vi "InitConfiguration.vi"(8 "error in":errorcluster) -> (0 "error out":errorcluster)   [LabVIEW 2012]
uses:
  <vilib>/Utility/config.llb/Read Key (U32).vi
  <vilib>/Utility/config.llb/Read Key (Double).vi
  GlobalVariables/GantnerParameters.vi
  <vilib>/Utility/config.llb/Read Key (String).vi
  GlobalVariables/PT02Parameters.vi
  GlobalVariables/PT03Parameters.vi
  <vilib>/Utility/config.llb/Read Key (I32).vi
  GlobalVariables/FT01Parameters.vi
  GlobalVariables/FT02Parameters.vi
  <vilib>/Utility/config.llb/Read Key (Boolean).vi
  GlobalVariables/SystemParameters.vi
  GlobalVariables/HardwarePresent.vi
  GlobalVariables/StabilizationSettings.vi
  <vilib>/Utility/config.llb/NI_LVConfig.lvlib
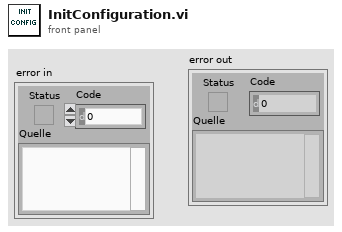
[diagram p1: front panel]
types:
  T1 = typedef "NI_LVConfig.lvlib/Config Data RefNum.ctl" = refnum<k1>
  T2 = typedef "ISMBUS_Module.ctl" = cluster{"ModuleAddress":i32, "ModuleKindIndex":i32, "ModuleKind":string, " Protocol":string, " BaudRate":i32, "CharFormat":string, "BaudRateIndex":i32, "FormatIndex":i32, "ProtocolIndex":i32, "Location":string, "SerialNumber":string, "Vendor":string, "HWRelease":string, "SWRelease":string, "ControllerType":string, "ChannelList":T3[], "ChannelCount":i32, " COM Port":i32}
  T3 = typedef "ISMBUS_Channel.ctl" = cluster{" Description":string, " ChannelKindIndex":i32, "ChannelFormatIndex":i32, " FieldLength":i32, "Precision":i32, "Unit":string, "Mode":i32}
  T4 = cluster{"Module":T2, "value":u32, "value":u32, "value":u32, "value":u32, "value":dbl}
  T5 = cluster{"value":u32, "value":string, "value":u32, "value":dbl, "value":u32}
  T6 = cluster{"value":u32, "value":i32, "value":i32, "value":dbl, "IDH":u8, "IDM":u8, "IDL":u8, "IDS":u8}
  T7 = cluster{"value":string, "value":string, "value":string, "value":bool}
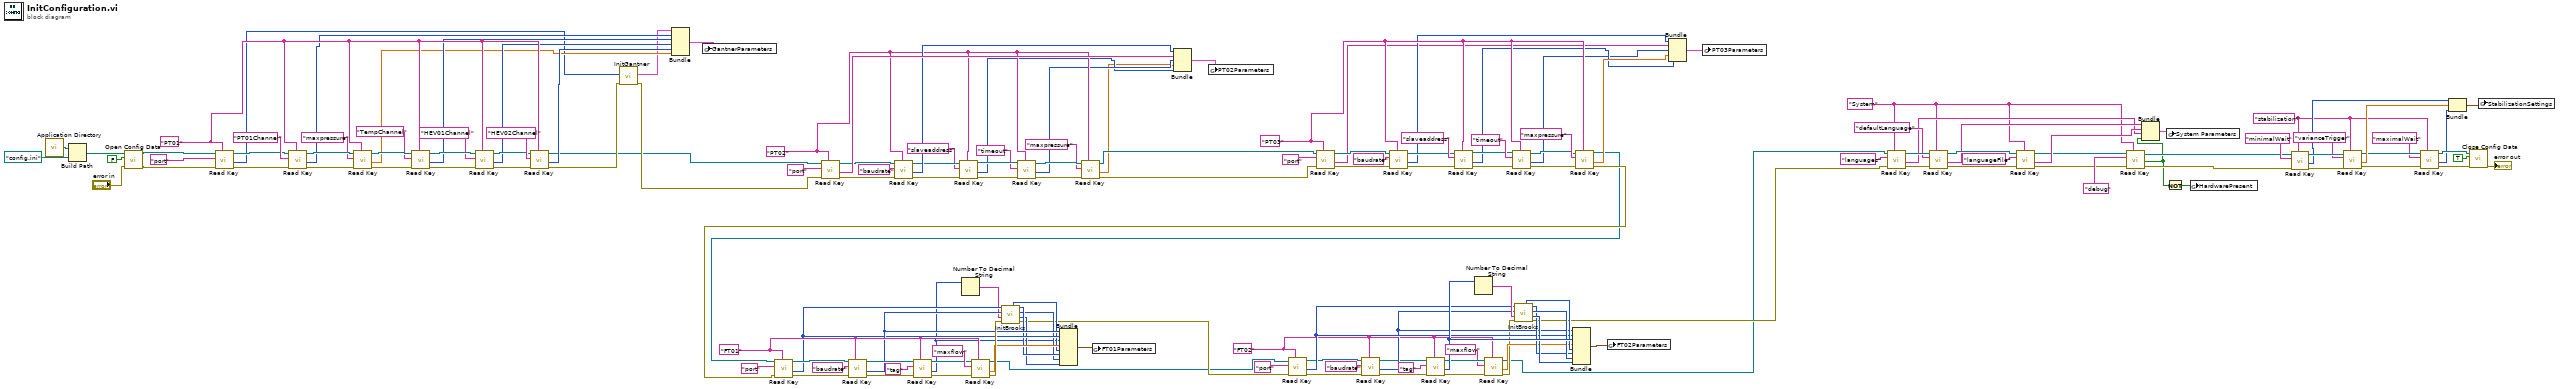
[diagram p0: block diagram]
diagram:
  w18 = "FT02" ("section")
  w40 = "FT01" ("section")
  w76 = "PT02" ("section")
  w108 = "PT01" ("section")
  w119 = "stabilization"
  w114 = "System" ("section")
  w124 = "PT03" ("section")
  n1 = call <vilib>:"Application Directory.vi"() -> ("Application Directory"=w158:path)
  n2 = Build Path(base path=w158, name or relative path=path "config.ini" ("default name")) -> (appended path=w159:path)
  n3 = call <vilib>:"Open Config Data.vi"("error in (no error)"="error in", "create file if necessary (T)"=FALSE ("create file if necessary? (T)"), "configuration file path"=w159) -> ("error out"=w89:errorcluster, "refnum"=w90:T1)  [unwired: 6 in, 1 out]
  n4 = call-poly <vilib>:"Read Key.vi"("section"=w108, "error in (no error)"=w89, "key"="port", "refnum"=w90) -> ("error out"=w102:errorcluster, "value"=w83:u32, "refnum out"=w103:T1)  [unwired: 4 in, 1 out]
  n5 = call-poly <vilib>:"Read Key.vi"("section"=w108, "error in (no error)"=w102, "key"="PT01Channel", "refnum"=w103) -> ("error out"=w107:errorcluster, "value"=w88:u32, "refnum out"=w106:T1)  [unwired: 4 in, 1 out]
  n6 = call-poly <vilib>:"Read Key.vi"("section"=w108, "error in (no error)"=w107, "key"="maxpressure", "refnum"=w106) -> ("error out"=w99:errorcluster, "value"=w84:dbl, "refnum out"=w100:T1)  [unwired: 4 in, 1 out]
  n7 = call-poly <vilib>:"Read Key.vi"("section"=w108, "error in (no error)"=w99, "key"="TempChannel", "refnum"=w100) -> ("error out"=w93:errorcluster, "value"=w87:u32, "refnum out"=w94:T1)  [unwired: 4 in, 1 out]
  n8 = call-poly <vilib>:"Read Key.vi"("section"=w108, "error in (no error)"=w93, "key"="HEV01Channel", "refnum"=w94) -> ("error out"=w95:errorcluster, "value"=w86:u32, "refnum out"=w96:T1)  [unwired: 4 in, 1 out]
  n9 = call-poly <vilib>:"Read Key.vi"("section"=w108, "error in (no error)"=w95, "key"="HEV02Channel", "refnum"=w96) -> ("error out"=w81:errorcluster, "value"=w85:u32, "refnum out"=w60:T1)  [unwired: 4 in, 1 out]
  n10 = call "InitGantner.vi"("error in"=w81, "Port"=w83) -> ("error out"=w61:errorcluster, "Module"=w82:T2)  [unwired: 8 in]
  n11 = Bundle("Module"=w82, "value"=w88, "value"=w87, "value"=w86, "value"=w85, "value"=w84) -> (w98:T4)  [unwired: 1 in]
  n12 = global write "GantnerParameters.vi" "GantnerParameters"(w98) -> ()
  n13 = call-poly <vilib>:"Read Key.vi"("section"=w76, "error in (no error)"=w61, "key"="port", "refnum"=w60) -> ("error out"=w70:errorcluster, "value"=w78:string, "refnum out"=w71:T1)  [unwired: 4 in, 1 out]
  n14 = call-poly <vilib>:"Read Key.vi"("section"=w76, "error in (no error)"=w70, "key"="baudrate", "refnum"=w71) -> ("error out"=w75:errorcluster, "value"=w77:u32, "refnum out"=w74:T1)  [unwired: 4 in, 1 out]
  n15 = call-poly <vilib>:"Read Key.vi"("section"=w76, "error in (no error)"=w75, "key"="slaveaddress", "refnum"=w74) -> ("error out"=w67:errorcluster, "value"=w55:u32, "refnum out"=w68:T1)  [unwired: 4 in, 1 out]
  n16 = call-poly <vilib>:"Read Key.vi"("section"=w76, "error in (no error)"=w67, "key"="timeout", "refnum"=w68) -> ("error out"=w64:errorcluster, "value"=w56:u32, "refnum out"=w65:T1)  [unwired: 4 in, 1 out]
  n17 = call-poly <vilib>:"Read Key.vi"("section"=w76, "error in (no error)"=w64, "key"="maxpressure", "refnum"=w65) -> ("error out"=w59:errorcluster, "value"=w54:dbl, "refnum out"=w58:T1)  [unwired: 4 in, 1 out]
  n18 = Bundle("value"=w77, "value"=w78, "value"=w56, "value"=w54, "value"=w55) -> (w66:T5)  [unwired: 1 in]
  n19 = global write "PT02Parameters.vi" "PT02Parameters"(w66) -> ()
  n20 = call-poly <vilib>:"Read Key.vi"("section"=w124, "error in (no error)"=w59, "key"="port", "refnum"=w58) -> ("error out"=w148:errorcluster, "value"=w79:string, "refnum out"=w147:T1)  [unwired: 4 in, 1 out]
  n21 = call-poly <vilib>:"Read Key.vi"("section"=w124, "error in (no error)"=w148, "key"="baudrate", "refnum"=w147) -> ("error out"=w143:errorcluster, "value"=w80:u32, "refnum out"=w144:T1)  [unwired: 4 in, 1 out]
  n22 = call-poly <vilib>:"Read Key.vi"("section"=w124, "error in (no error)"=w143, "key"="slaveaddress", "refnum"=w144) -> ("error out"=w151:errorcluster, "value"=w52:u32, "refnum out"=w150:T1)  [unwired: 4 in, 1 out]
  n23 = call-poly <vilib>:"Read Key.vi"("section"=w124, "error in (no error)"=w151, "key"="timeout", "refnum"=w150) -> ("error out"=w154:errorcluster, "value"=w51:u32, "refnum out"=w153:T1)  [unwired: 4 in, 1 out]
  n24 = call-poly <vilib>:"Read Key.vi"("section"=w124, "error in (no error)"=w154, "key"="maxpressure", "refnum"=w153) -> ("error out"=w6:errorcluster, "value"=w53:dbl, "refnum out"=w5:T1)  [unwired: 4 in, 1 out]
  n25 = call-poly <vilib>:"Read Key.vi"("section"=w40, "error in (no error)"=w6, "key"="port", "refnum"=w5) -> ("error out"=w46:errorcluster, "value"=w37:i32, "refnum out"=w45:T1)  [unwired: 4 in, 1 out]
  n26 = call-poly <vilib>:"Read Key.vi"("section"=w40, "error in (no error)"=w46, "key"="baudrate", "refnum"=w45) -> ("error out"=w41:errorcluster, "value"=w38:u32, "refnum out"=w42:T1)  [unwired: 4 in, 1 out]
  n27 = call-poly <vilib>:"Read Key.vi"("section"=w40, "error in (no error)"=w41, "key"="tag", "refnum"=w42) -> ("error out"=w49:errorcluster, "value"=w30:i32, "refnum out"=w48:T1)  [unwired: 4 in, 1 out]
  n28 = Number To Decimal String(number=w30) -> (decimal integer string=w29:string)  [unwired: 1 in]
  n29 = call-poly <vilib>:"Read Key.vi"("section"=w40, "error in (no error)"=w49, "key"="maxflow", "refnum"=w48) -> ("error out"=w39:errorcluster, "value"=w36:dbl, "refnum out"=w3:T1)  [unwired: 4 in, 1 out]
  n30 = call "InitBrooks.vi"("error in"=w39, "TAG"=w29, "Baud"=w38, "COM"=w37) -> ("error out"=w4:errorcluster, "IDS"=w32:u8, "IDL"=w33:u8, "IDM"=w34:u8, "IDH"=w35:u8)  [unwired: 3 in]
  n31 = Bundle("value"=w38, "value"=w37, "value"=w30, "value"=w36, "IDH"=w35, "IDM"=w34, "IDL"=w33, "IDS"=w32) -> (w31:T6)  [unwired: 1 in]
  n32 = global write "FT01Parameters.vi" "FT01Parameters"(w31) -> ()
  n33 = call-poly <vilib>:"Read Key.vi"("section"=w18, "error in (no error)"=w4, "key"="port", "refnum"=w3) -> ("error out"=w12:errorcluster, "value"=w21:i32, "refnum out"=w13:T1)  [unwired: 4 in, 1 out]
  n34 = call-poly <vilib>:"Read Key.vi"("section"=w18, "error in (no error)"=w12, "key"="baudrate", "refnum"=w13) -> ("error out"=w17:errorcluster, "value"=w20:u32, "refnum out"=w16:T1)  [unwired: 4 in, 1 out]
  n35 = call-poly <vilib>:"Read Key.vi"("section"=w18, "error in (no error)"=w17, "key"="tag", "refnum"=w16) -> ("error out"=w9:errorcluster, "value"=w27:i32, "refnum out"=w10:T1)  [unwired: 4 in, 1 out]
  n36 = Number To Decimal String(number=w27) -> (decimal integer string=w28:string)  [unwired: 1 in]
  n37 = call-poly <vilib>:"Read Key.vi"("section"=w18, "error in (no error)"=w9, "key"="maxflow", "refnum"=w10) -> ("error out"=w19:errorcluster, "value"=w22:dbl, "refnum out"=w1:T1)  [unwired: 4 in, 1 out]
  n38 = call "InitBrooks.vi"("error in"=w19, "TAG"=w28, "Baud"=w20, "COM"=w21) -> ("error out"=w2:errorcluster, "IDS"=w26:u8, "IDL"=w25:u8, "IDM"=w24:u8, "IDH"=w23:u8)  [unwired: 3 in]
  n39 = Bundle("value"=w20, "value"=w21, "value"=w27, "value"=w22, "IDH"=w23, "IDM"=w24, "IDL"=w25, "IDS"=w26) -> (w7:T6)  [unwired: 1 in]
  n40 = global write "FT02Parameters.vi" "FT02Parameters"(w7) -> ()
  n41 = Bundle("value"=w80, "value"=w79, "value"=w51, "value"=w53, "value"=w52) -> (w57:T5)  [unwired: 1 in]
  n42 = global write "PT03Parameters.vi" "PT03Parameters"(w57) -> ()
  n43 = call-poly <vilib>:"Read Key.vi"("section"=w114, "error in (no error)"=w2, "key"="languages" ("section"), "refnum"=w1) -> ("error out"=w139:errorcluster, "value"=w133:string, "refnum out"=w142:T1)  [unwired: 4 in, 1 out]
  n44 = call-poly <vilib>:"Read Key.vi"("section"=w114, "error in (no error)"=w139, "key"="defaultLanguage" ("section"), "refnum"=w142) -> ("error out"=w140:errorcluster, "value"=w135:string, "refnum out"=w141:T1)  [unwired: 4 in, 1 out]
  n45 = call-poly <vilib>:"Read Key.vi"("section"=w114, "error in (no error)"=w140, "key"="languageFile" ("section"), "refnum"=w141) -> ("error out"=w111:errorcluster, "value"=w134:string, "refnum out"=w109:T1)  [unwired: 4 in, 1 out]
  n46 = call-poly <vilib>:"Read Key.vi"("section"=w114, "error in (no error)"=w111, "key"="debug", "refnum"=w109) -> ("error out"=w115:errorcluster, "value"=w110:bool, "refnum out"=w116:T1)  [unwired: 4 in, 1 out]
  n47 = Bundle("value"=w135, "value"=w134, "value"=w133, "value"=w110) -> (w132:T7)  [unwired: 1 in]
  n48 = global write "SystemParameters.vi" "System Parameters"(w132) -> ()
  n49 = Not(x=w110) -> (.not. x?=w112:bool)
  n50 = global write "HardwarePresent.vi" "HardwarePresent"(w112) -> ()
  n51 = call-poly <vilib>:"Read Key.vi"("section"=w119, "error in (no error)"=w115, "key"="minimalWait", "refnum"=w116) -> ("error out"=w131:errorcluster, "value"=w126:u32, "refnum out"=w130:T1)  [unwired: 4 in, 1 out]
  n52 = call-poly <vilib>:"Read Key.vi"("section"=w119, "error in (no error)"=w131, "key"="varianceTrigger", "refnum"=w130) -> ("error out"=w120:errorcluster, "value"=w125:dbl, "refnum out"=w123:T1)  [unwired: 4 in, 1 out]
  n53 = call-poly <vilib>:"Read Key.vi"("section"=w119, "error in (no error)"=w120, "key"="maximalWait", "refnum"=w123) -> ("error out"=w121:errorcluster, "value"=w117:u32, "refnum out"=w122:T1)  [unwired: 4 in, 1 out]
  n54 = Bundle("value"=w126, "value"=w125, "value"=w117) -> (w127:cluster{"value":u32, "value":dbl, "value":u32})  [unwired: 1 in]
  n55 = call <vilib>:"Close Config Data.vi"("error in (no error)"=w121, "write file if changed (T)"=TRUE ("write configuration file? (T)"), "refnum"=w122) -> ("error out"=→"error out":errorcluster)  [unwired: 8 out]
  n56 = global write "StabilizationSettings.vi" "StabilizationSettings"(w127) -> ()
